vi "unormalizada.vi"(11 "upq":T1) -> (3 "x/y":i32)   [LabVIEW 2021]
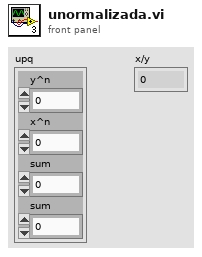
[diagram p1: front panel]
types:
  T1 = cluster{"y^n":dbl, "x^n":dbl, "sum":dbl, "sum":dbl}
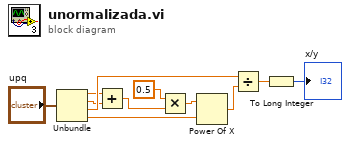
[diagram p0: block diagram]
diagram:
  n1 = Unbundle("upq") -> ("y^n"=w3:dbl, "x^n"=w4:dbl, "sum"=w9:dbl, "sum"=w8:dbl)
  n2 = Add(x=w3, y=w4) -> (x+y=w5:dbl)
  n3 = Multiply(x=0.5, y=w5) -> (x*y=w7:dbl)
  n4 = Power Of X(1:w8, 2:w7) -> (0:w10:dbl)
  n5 = Divide(x=w9, y=w10) -> (x/y=w2:dbl)
  n6 = To Long Integer(number=w2) -> (32bit integer=→"x/y":i32)
